vi "Execute Previous Command.vi"(8 "error in (no error)":errorcluster, 10 "index":i32, 11 "Command Handler in":refnum<class "Command Handler.lvclass">) -> (0 "error out":errorcluster, 3 "Command Handler out":refnum<class "Command Handler.lvclass">)   [LabVIEW 2017, in "Command Handler.lvlib" / "Command Handler.lvclass"]
uses:
  Command Handler.lvclass
  Command Handler.lvclass/Command Handler.ctl
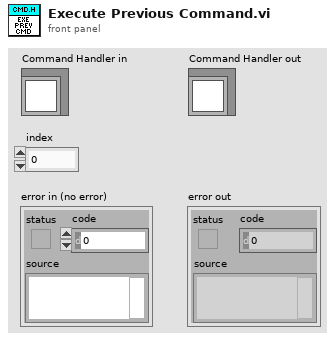
[diagram p1: front panel]
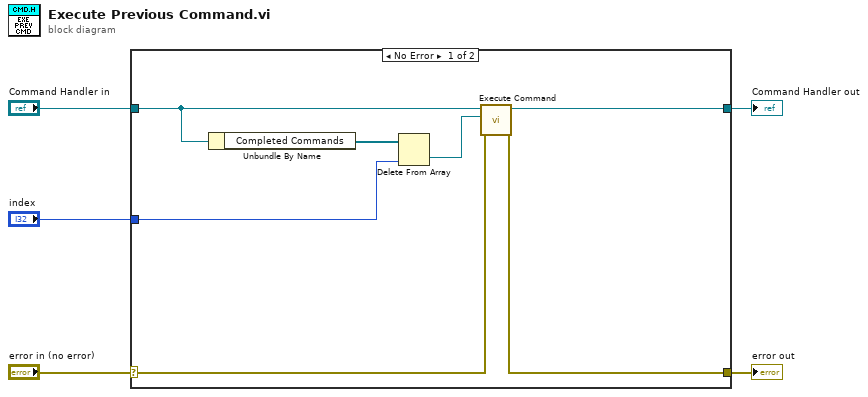
[diagram p0: block diagram]
diagram:
  n1 = case shown="No Error" "error in (no error)" {
    selector: "error in (no error)" -> [w9 w14]
    tunnel: [w8 w14] -> w4
    tunnel: [w10 w13] -> w2
    tunnel: "Command Handler in" -> [w11 w13]
    tunnel: "index" -> [w6 _]
    frame No Error {
      n2 = Unbundle By Name(w11) -> ("Completed Commands"=w12:refnum<class "Command.lvclass">[])
      n3 = Delete From Array(array=w12, index=w6) -> (deleted portion=w7:refnum<class "Command.lvclass">)  [unwired: 1 in, 1 out]
      n4 = call-dynamic "Execute Command.vi"("error in (no error)"=w9, "Command"=w7, "Command Handler in"=w11) -> ("error out"=w8:errorcluster, "Command Handler out"=w10:refnum<class "Command Handler.lvclass">)  [unwired: 6 in, 1 out]
    }
    frame Error {
    }
  }
  "error out" <- w4
  "Command Handler out" <- w2
